vi "onStart.vi"(8 "error in (no error)":errorcluster, 11 "Inst.Transport":refnum<class "Inst.Transport.lvclass">) -> (0 "error out":errorcluster, 3 "Inst.Transport out":refnum<class "Inst.Transport.lvclass">)   [LabVIEW 2019, in "Inst.Transport.lvclass"]
uses:
  Inst.Transport.lvclass
  Typedefs/Inst.Transport.Status--Enum.ctl
  Inst.Transport.lvclass/Inst.Transport.ctl
  Transport/Transport.lvclass/Transport.ctl
  <userlib>/LevyLab/Instrument Framework/Instrument Types/SCPI/Instrument.SCPI.lvclass
  Transport/Transport.lvclass
panel:
  # "For instructions on how to use the JKI State Machine Objects, examples and video tutorials, visit:\nhttp://jki.net/state-machine-objects/\n\nJKI State Machine Objects™\nhttp://jki.net/state-machine-objects/\nCopyright (C) 2005-2015, JKI <info@jki.net>\nALL RIGHTS RESERVED"
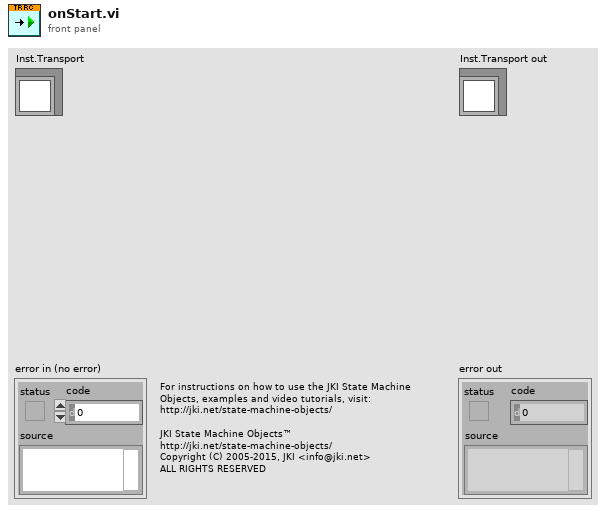
[diagram p1: front panel]
types:
  T1 = typedef "Inst.Transport.lvclass/Inst.Transport.Status--Enum.ctl" = enum16{"idle", "running"}
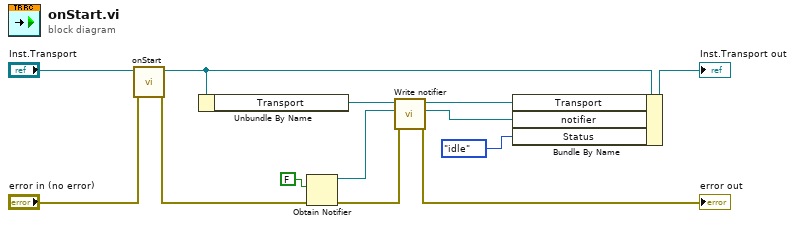
[diagram p0: block diagram]
diagram:
  n1 = call-parent "onStart.vi"("error in (no error)"="error in (no error)", "SMO"="Inst.Transport") -> ("error out"=w6:errorcluster, "SMO out"=w3:refnum<class "Inst.Transport.lvclass">)  [unwired: 8 in]
  n2 = Unbundle By Name(w3) -> ("Transport"=w9:refnum<class "Transport.lvclass">)
  n3 = Obtain Notifier(notification data type=FALSE, error in (no error)=w6) -> (notifier out=w2:refnum<notifier>, error out=w5:errorcluster)  [unwired: 2 in, 1 out]
  n4 = call "Write notifier.vi"("error in (no error)"=w5, "notifier"=w2, "Transport in"=w9) -> ("error out"=→"error out":errorcluster, "Transport out"=w10:refnum<class "Transport.lvclass">)  [unwired: 7 in]
  n5 = Bundle By Name(cluster=w3, "Transport"=w10, "notifier"=w2, "Status"=Inst.Transport.Status--Enum."idle") -> (→"Inst.Transport out":refnum<class "Inst.Transport.lvclass">)
